vi "DB_Main.vi"   [LabVIEW 2017, in "Dashboard.lvlib"]
uses:
  Dashboard.lvlib
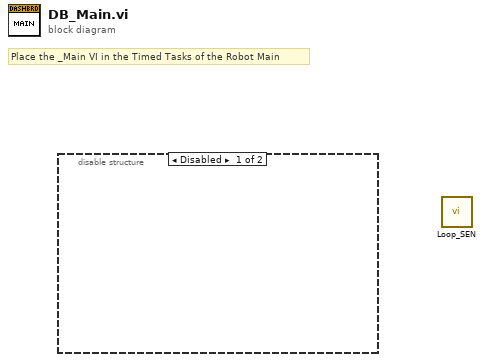
[diagram p0: block diagram]
diagram:
  # "Place the _Main VI in the Timed Tasks of the Robot Main"
  n1 = disable-structure shown="Disabled" {
    frame Disabled {
    }
    frame Enabled {
    }
  }
  n2 = call "Loop_SEN.vi"() -> ()  [unwired: 12 in]
